vi "log_acquisition.vi"(1 "log_data":T1) -> (0 "Log":string)   [LabVIEW 2016]
uses:
  log_data.ctl
  log_status.ctl
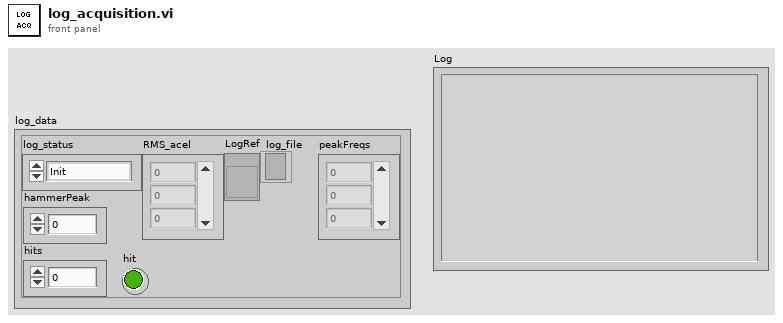
[diagram p1: front panel]
types:
  T1 = typedef "log_data.ctl" = cluster{"log_status":T2, "RMS_acel":dbl[], "LogRef":refnum<vi>, "log_file":refnum<file>, "hammerPeak":dbl, "peakFreqs":dbl[], "hits":i32, "hit":bool}
  T2 = typedef "log_status.ctl" = enum16{"Init", "Ready", "Running", "Error", "End"}
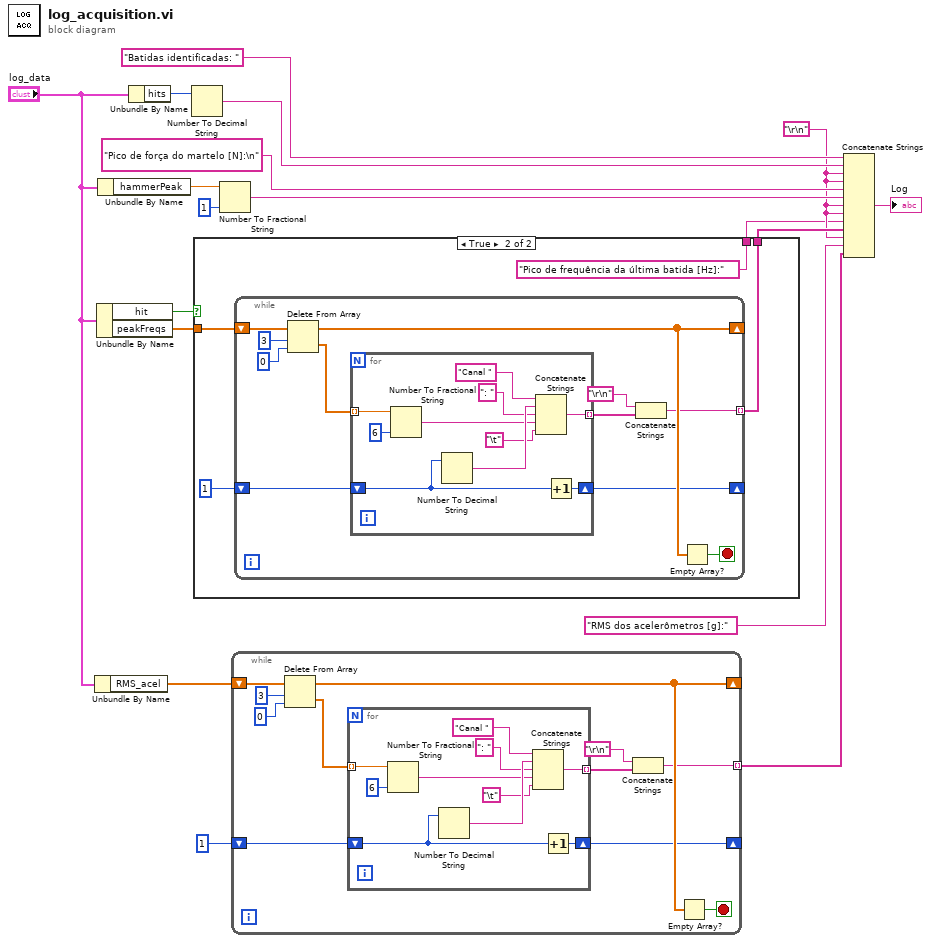
[diagram p0: block diagram]
diagram:
  w4 = "\r\n"
  n1 = Unbundle By Name("log_data") -> ("RMS_acel"=w10:dbl[])
  n2 = Unbundle By Name("log_data") -> ("hit"=w1:bool, "peakFreqs"=w18:dbl[])
  n3 = Unbundle By Name("log_data") -> ("hammerPeak"=w14:dbl)
  n4 = Unbundle By Name("log_data") -> ("hits"=w7:i32)
  n5 = Number To Decimal String(number=w7) -> (decimal integer string=w6:string)  [unwired: 1 in]
  n6 = case shown="True" w1 {
    tunnel: w18 -> [_ w22]
    tunnel: [_ w20] -> w17
    tunnel: [_ "Pico de frequência da última batida [Hz]:" ("string")] -> w3
    frame False {
    }
    frame True {
      n7 = while {
        shift-right: [w30] -> _
        shift-left: w22 -> [w33]
        shift-right: [w26] -> _
        shift-left: i16 1 ("precision (6)") -> [w27]
        tunnel: [w23] -> w20 mode=indexing
        stop <- w29 stop-if-true
        n8 = Delete From Array(array=w33, length=3, index=0) -> (deleted portion=w28:dbl[], array with subset deleted=w30:dbl[])
        n9 = for {
          tunnel: w28 -> [w43] mode=indexing
          shift-right: [w41] -> w26
          shift-left: w27 -> [w40]
          tunnel: [w35] -> w25 mode=indexing
          n10 = Number To Fractional String(number=w43, precision (6)=i16 6) -> (F-format string=w36:string)  [unwired: 2 in]
          n11 = Number To Decimal String(number=w40) -> (decimal integer string=w39:string)  [unwired: 1 in]
          n12 = Concatenate Strings("Canal " ("string"), w39, ": " ("string"), w36, "\t") -> (w35:string)
          n13 = Increment(x=w40) -> (x+1=w41:i16)
        }
        n14 = Concatenate Strings("\r\n", w25) -> (w23:string)
        n15 = Empty Array?(array=w30) -> (empty?=w29:bool)
      }
    }
  }
  n16 = Number To Fractional String(number=w14, precision (6)=i16 1) -> (F-format string=w13:string)  [unwired: 2 in]
  n17 = while {
    shift-right: [w51] -> _
    shift-left: w10 -> [w54]
    shift-right: [w47] -> _
    shift-left: i16 1 ("precision (6)") -> [w48]
    tunnel: [w44] -> w9 mode=indexing
    stop <- w50 stop-if-true
    n18 = Delete From Array(array=w54, length=3, index=0) -> (deleted portion=w49:dbl[], array with subset deleted=w51:dbl[])
    n19 = for {
      tunnel: w49 -> [w64] mode=indexing
      shift-right: [w62] -> w47
      shift-left: w48 -> [w61]
      tunnel: [w56] -> w46 mode=indexing
      n20 = Number To Fractional String(number=w64, precision (6)=i16 6) -> (F-format string=w57:string)  [unwired: 2 in]
      n21 = Number To Decimal String(number=w61) -> (decimal integer string=w60:string)  [unwired: 1 in]
      n22 = Concatenate Strings("Canal " ("string"), w60, ": " ("string"), w57, "\t") -> (w56:string)
      n23 = Increment(x=w61) -> (x+1=w62:i16)
    }
    n24 = Concatenate Strings("\r\n", w46) -> (w44:string)
    n25 = Empty Array?(array=w51) -> (empty?=w50:bool)
  }
  n26 = Concatenate Strings("Batidas identificadas: " ("string"), w6, w4, w4, "Pico de força do martelo [N]:\n" ("string"), w13, w4, w4, w3, w17, w4, "RMS dos acelerômetros [g]:" ("string"), w9) -> (→"Log":string)
